vi "view curr alr state_2.vi"(6 "ALR_Descriptions":string[](array[string]), 9 "ALR_Names":string[](array[string]), 10 "ALR_State":T1, 11 "Alarms Listbox":refnum<vi>) -> ()   [LabVIEW 2019, in "Alarms.lvlib"]
uses:
  Alarms.lvlib
  Ctl/ALRs_State.ctl
  <vilib>/Utility/miscctls.llb/LVRowAndColumnTypeDef.ctl
  Userlib.lvlib
  Logik/Logik.lvlib
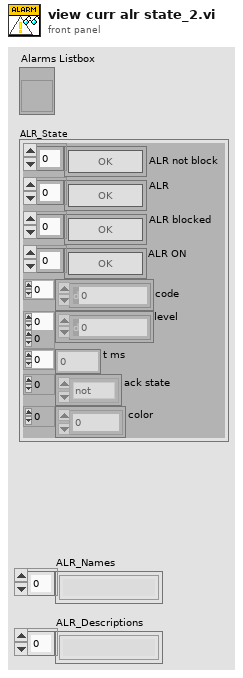
[diagram p1: front panel]
types:
  T1 = typedef "Alarms.lvlib/ALRs_State.ctl" = cluster{"ALR not block":bool[], "ALR":bool[], "ALR blocked":bool[], "ALR ON":bool[], "code":i32[], "level":i32[][], "t ms":u32[], "ack state":enum32{"not", "tripped", "reset", "ack"}[], "color":u32[]}
  T2 = typedef "LVRowAndColumnTypeDef.ctl" = cluster{"Row":i32, "Column":i32}
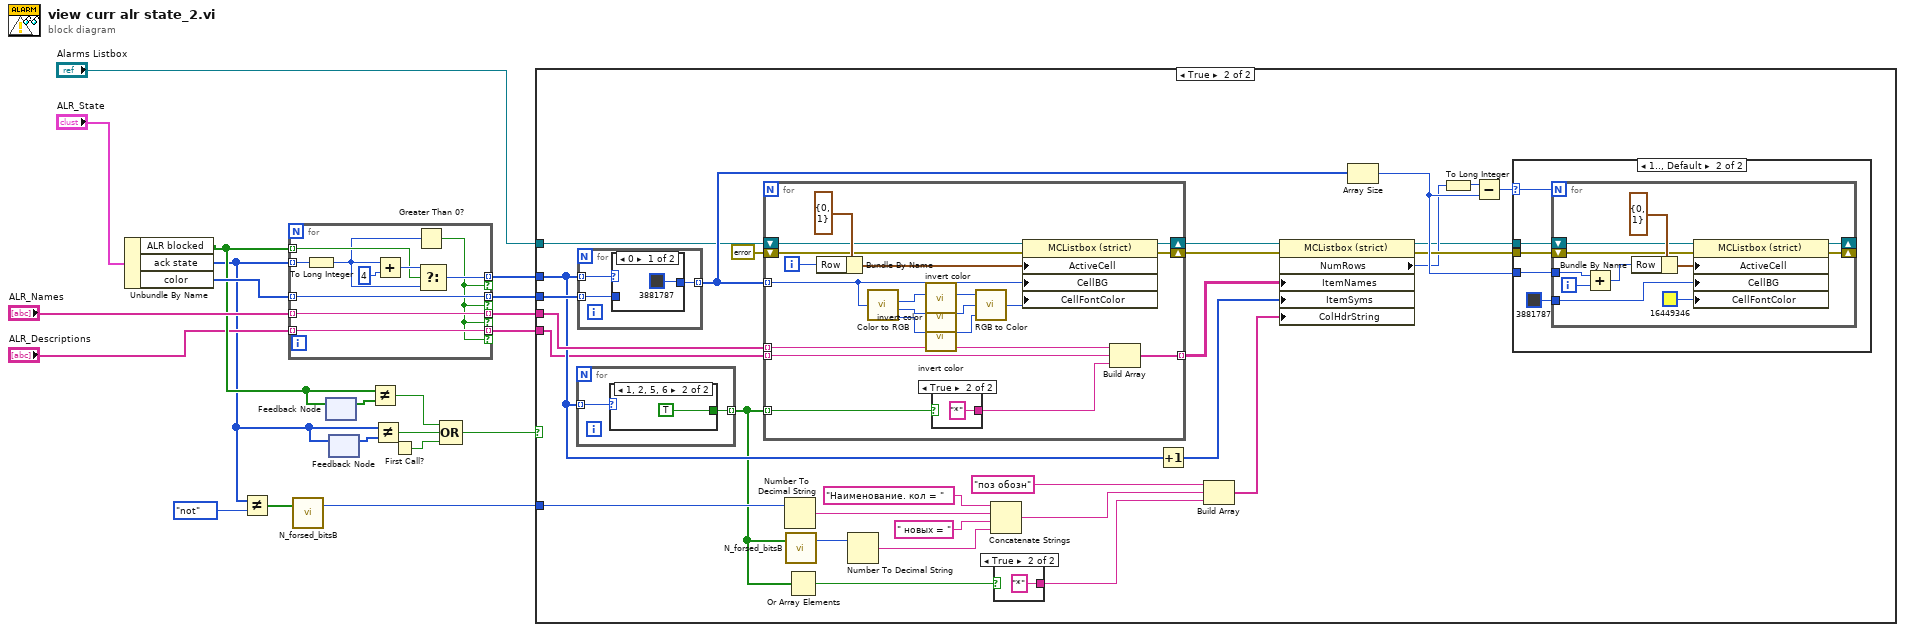
[diagram p0: block diagram]
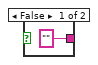
[diagram p3: hidden frame]
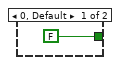
[diagram p6: hidden frame]
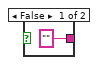
[diagram p7: hidden frame]
diagram:
  n1 = Unbundle By Name("ALR_State") -> ("ALR blocked"=w8:bool[], "ack state"=w2:enum32{"not", "tripped", "reset", "ack"}[], "color"=w14:u32[])
  n2 = Not Equal?(x=w2, y=enum32{"not", "tripped", "reset", "ack"}."not" ("ack state")) -> (x != y?=w4:bool[])
  n3 = for {
    tunnel: [w30] -> w16 mode=indexing if=w21
    tunnel: [w26] -> w15 mode=indexing if=w21
    tunnel: [w25] -> w18 mode=indexing if=w21
    tunnel: w2 -> [w27] mode=indexing
    tunnel: w14 -> [w26] mode=indexing
    tunnel: "ALR_Names" -> [w25] mode=indexing
    tunnel: w8 -> [w24] mode=indexing
    tunnel: "ALR_Descriptions" -> [w22] mode=indexing
    tunnel: [w22] -> w5 mode=indexing if=w21
    n4 = To Long Integer(number=w27) -> (32bit integer=w23:i32)
    n5 = Add(x=w23, y=4) -> (x+y=w28:i32)
    n6 = Greater Than 0?(x=w23) -> (x > 0?=w21:bool)
    n7 = Select(t=w28, s=w24, f=w23) -> (s? t:f=w30:i32)
  }
  n8 = call "N_forsed_bitsB.vi"("IN"=w4) -> ("N_forsed_bits"=w3:i32)  [unwired: 2 in]
  n9 = feedback #1() -> (w11:bool[])  [unwired: 1 in]
  n10 = feedback-in #1(w8) -> ()
  n11 = feedback #2() -> (w13:enum32{"not", "tripped", "reset", "ack"}[])  [unwired: 1 in]
  n12 = feedback-in #2(w2) -> ()
  n13 = Not Equal?(x=w8, y=w11) -> (x != y?=w9:bool)
  n14 = Not Equal?(x=w2, y=w13) -> (x != y?=w12:bool)
  n15 = First Call?() -> (First Call?: T/F=w7:bool)
  n16 = Compound Arithmetic op=OR(w9, w12, w7) -> (w17:bool)
  n17 = case shown="True" w17 {
    tunnel: w18 -> [_ w59]
    tunnel: w16 -> [_ w56]
    tunnel: w15 -> [_ w58]
    tunnel: "Alarms Listbox" -> [_ w46]
    tunnel: w5 -> [_ w43]
    tunnel: w3 -> [_ w42]
    frame False {
    }
    frame True {
      n18 = for {
        tunnel: [w84] -> w32 mode=indexing
        tunnel: w56 -> [w83] mode=indexing
        n19 = case shown="1, 2, 5, 6" w83 {
          tunnel: [FALSE TRUE] -> w84
          frame 0, Default {
          }
          frame 1, 2, 5, 6 {
          }
        }
      }
      n20 = for {
        tunnel: w56 -> [w79] mode=indexing
        tunnel: [w80] -> w55 mode=indexing
        tunnel: w58 -> [w78] mode=indexing
        n21 = case shown="0" w79 {
          tunnel: [u32 3881787 w82] -> w80
          tunnel: w78 -> [_ w82]
          frame 0 {
          }
          frame 1, Default {
          }
        }
      }
      n22 = for {
        tunnel: w55 -> [w100] mode=indexing
        tunnel: w32 -> [w104] mode=indexing
        tunnel: w59 -> [w88] mode=indexing
        tunnel: [w101] -> w57 mode=indexing
        shift-right: [w92] -> w51
        shift-left: errorcluster {"status"=FALSE, "code"=0, "source"=""} ("error out") -> [w91]
        shift-right: [w89] -> w45
        shift-left: w46 -> [w90]
        tunnel: w43 -> [w87] mode=indexing
        i -> [w103]
        n23 = Bundle By Name(cluster=T2 {"Row"=0, "Column"=1} ("Active Cell:Active Cell"), "Row"=w103) -> (w105:T2)
        n24 = call <vilib>:"Color to RGB.vi"("Color"=w100) -> ("R"=w98:u8, "G"=w96:u8, "B"=w93:u8)  [unwired: 1 out]
        n25 = call "invert color.vi"("color"=w98) -> ("invert color"=w97:u8)  [unwired: 10 in]
        n26 = call "invert color.vi"("color"=w96) -> ("invert color"=w95:u8)  [unwired: 10 in]
        n27 = call "invert color.vi"("color"=w93) -> ("invert color"=w94:u8)  [unwired: 10 in]
        n28 = case shown="True" w104 {
          tunnel: ["" ("Caption.Text") "*" ("Caption.Text")] -> w102
          frame False {
          }
          frame True {
          }
        }
        n29 = call <vilib>:"RGB to Color.vi"("B"=w94, "G"=w95, "R"=w97) -> ("Color"=w99:u32)
        n30 = property on="Property Node" class="MCListbox (strict)"(reference=w90, error in=w91, "ActiveCell"=w105, "CellBG"=w100, "CellFontColor"=w99) -> (reference out=w89:refnum<vi>, error out=w92:errorcluster)
        n31 = Build Array(w88, w87, w102) -> (w101:string[])
      }
      n32 = Number To Decimal String(number=w42) -> (decimal integer string=w40:string)  [unwired: 1 in]
      n33 = call "N_forsed_bitsB.vi"("IN"=w32) -> ("N_forsed_bits"=w31:i32)  [unwired: 2 in]
      n34 = Or Array Elements(Boolean array=w32) -> (logical OR=w37:bool)
      n35 = Number To Decimal String(number=w31) -> (decimal integer string=w33:string)  [unwired: 1 in]
      n36 = Concatenate Strings("Наименование. кол = " ("Caption.Text"), w40, " новых = " ("Caption.Text"), w33) -> (w38:string)
      n37 = case shown="True" w37 {
        tunnel: ["" ("Caption.Text") "*" ("Caption.Text")] -> w36
        frame False {
        }
        frame True {
        }
      }
      n38 = Increment(x=w56) -> (x+1=w48:i32[])
      n39 = Build Array("поз обозн" ("Caption.Text"), w38, w36) -> (w34:string[])
      n40 = property on="Property Node" class="MCListbox (strict)"(reference=w45, error in=w51, "ItemNames"=w57, "ItemSyms"=w48, "ColHdrString"=w34) -> (reference out=w44:refnum<vi>, error out=w50:errorcluster, "NumRows"=w49:u32)
      n41 = Array Size(array=w55) -> (size(s)=w52:i32)
      n42 = To Long Integer(number=w49) -> (32bit integer=w54:i32)
      n43 = Subtract(x=w54, y=w52) -> (x-y=w53:i32)
      n44 = case shown="1.., Default" w53 {
        selector: w53 -> [_ w65]
        tunnel: w52 -> [_ w64]
        tunnel: w50 -> [_ w63]
        tunnel: w44 -> [_ w62]
        frame ..0 {
        }
        frame 1.., Default {
          n45 = for {
            N: w65 -> [_]
            tunnel: u32 3881787 -> [w75]
            shift-right: [w73] -> _
            shift-left: w63 -> [w74]
            tunnel: w64 -> [w70]
            shift-right: [w67] -> _
            shift-left: w62 -> [w68]
            i -> [w71]
            n46 = Add(x=w70, y=w71) -> (x+y=w69:i32)
            n47 = Bundle By Name(cluster=T2 {"Row"=0, "Column"=1} ("Active Cell:Active Cell"), "Row"=w69) -> (w76:T2)
            n48 = property on="Property Node" class="MCListbox (strict)"(reference=w68, error in=w74, "ActiveCell"=w76, "CellBG"=w75, "CellFontColor"=u32 16449346) -> (reference out=w67:refnum<vi>, error out=w73:errorcluster)
          }
        }
      }
    }
  }
